vi "Delete Scripting API.vi"(11 "Arguments":string[](array[string])) -> (2 "Output/Failure Message":string, 3 "Exit Code":i32)   [LabVIEW 2019]
panel:
  out "error out":errorcluster
  in  "error in":errorcluster
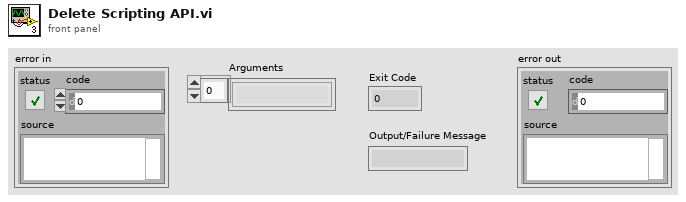
[diagram p1: front panel]
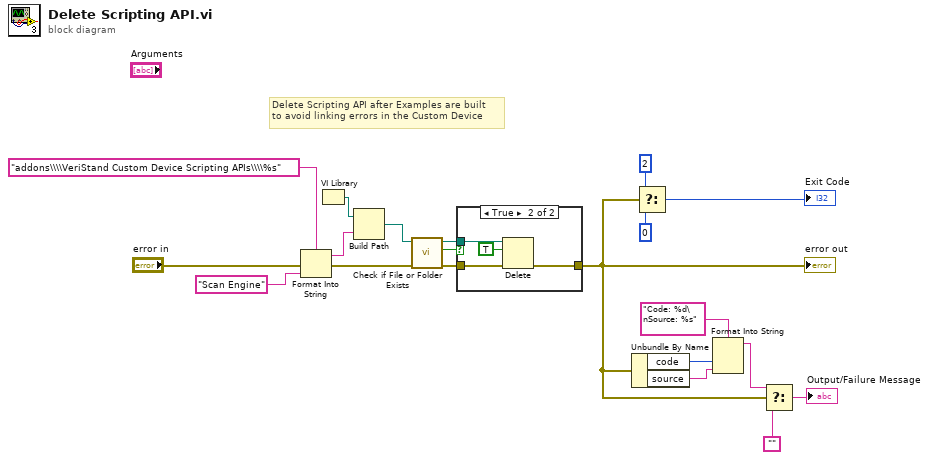
[diagram p0: block diagram]
diagram:
  # "Delete Scripting API after Examples are built\nto avoid linking errors in the Custom Device"
  n1 = Format Into String(format string="addons\\\\VeriStand Custom Device Scripting APIs\\\\%s" ("name or relative path"), error in="error in", "Scan Engine" ("CD Name")) -> (resulting string=w17:string, error out=w12:errorcluster)  [unwired: 1 in]
  n2 = VI Library() -> (path=w14:path)
  n3 = Build Path(base path=w14, name or relative path=w17) -> (appended path=w15:path)
  n4 = call <vilib>:"Check if File or Folder Exists.vi"("error in (no error)"=w12, "path"=w15) -> ("error out"=w18:errorcluster, "file or folder exists?"=w20:bool, "dup path"=w19:path)  [unwired: 7 in]
  n5 = case shown="True" w20 {
    tunnel: w19 -> [_ w25]
    tunnel: w18 -> [w21 w23]
    tunnel: [w21 w22] -> w1
    frame False {
    }
    frame True {
      n6 = Delete(path (use dialog)=w25, entire hierarchy (F)=TRUE, error in=w23) -> (error out=w22:errorcluster)  [unwired: 2 in, 2 out]
    }
  }
  "error out" <- w1
  n7 = Unbundle By Name(w1) -> ("code"=w8:i32, "source"=w7:string)
  n8 = Select(t=2 ("Exit Code"), s=w1, f=0 ("Exit Code")) -> (s? t:f=→"Exit Code":i32)
  n9 = Format Into String(format string="Code: %d\nSource: %s", w8, w7) -> (resulting string=w6:string)  [unwired: 2 in, 1 out]
  n10 = Select(t=w6, s=w1, f="") -> (s? t:f=→"Output/Failure Message":string)
